vi "getSuperKInfo.vi"(8 "error in (no error)":errorcluster, 11 "COMport":string="COM6") -> (0 "error out":errorcluster, 1 "extendedVersionInfo":string, 2 "firmwareVersion":u16, 4 "moduleType":i32 format="%x", 5 "moduleSerialNumber":string)   [LabVIEW 2015]
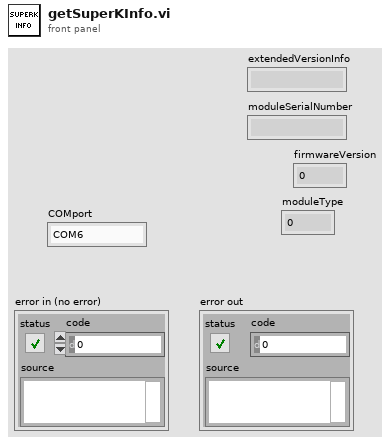
[diagram p1: front panel]
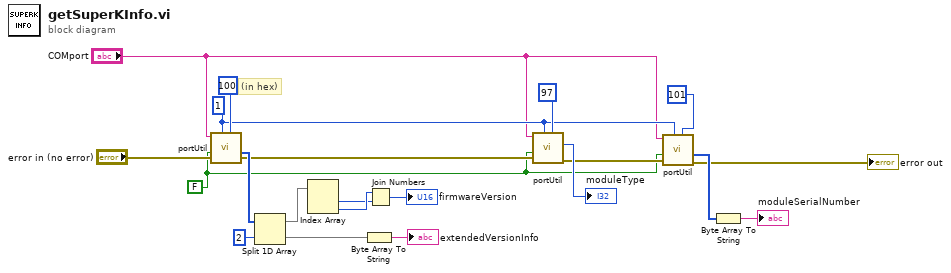
[diagram p0: block diagram]
diagram:
  w2 = FALSE ("WriteNotRead")
  w3 = u8 1 ("Destination")
  # "(in hex)"
  n1 = call "portUtil.vi"("Register"=u8 100, "Destination"=w3, "error in (no error)"="error in (no error)", "WriteNotRead"=w2, "COMport"="COMport") -> ("error out"=w9:errorcluster, "PayloadByteArray"=w20:u8[])  [unwired: 4 in, 1 out]
  n2 = Split 1D Array(array=w20, index=2) -> (first subarray=w17:u8[], second subarray=w15:u8[])
  n3 = Index Array(array=w17) -> (element #1=w18:u8, element #2=w19:u8)  [unwired: 2 in]
  n4 = Byte Array To String(unsigned byte array=w15) -> (string=→"extendedVersionInfo":string)
  n5 = Join Numbers(hi=w19, lo=w18) -> ((hi.lo)=→"firmwareVersion":u16)
  n6 = call "portUtil.vi"("Register"=u8 97, "Destination"=w3, "error in (no error)"=w9, "WriteNotRead"=w2, "COMport"="COMport") -> ("error out"=w6:errorcluster, "Long"=→"moduleType":i32)  [unwired: 4 in, 1 out]
  n7 = call "portUtil.vi"("Register"=u8 101, "Destination"=w3, "error in (no error)"=w6, "WriteNotRead"=w2, "COMport"="COMport") -> ("error out"=→"error out":errorcluster, "PayloadByteArray"=w8:u8[])  [unwired: 4 in, 1 out]
  n8 = Byte Array To String(unsigned byte array=w8) -> (string=→"moduleSerialNumber":string)
